vi "MB Slave Write Coils (poly).vi"(1 "Starting Address":u16, 2 "Coils":bool[](array[boolean]), 5 "error in":errorcluster) -> (19 "error out":errorcluster)   [LabVIEW 2023, in "Voegtlin_NI_SMART_Modbus_Drivers.lvlib"]
doc: "Writes multiple coils to the slave memory tables."
uses:
  Voegtlin_NI_SMART_Modbus_Drivers.lvlib
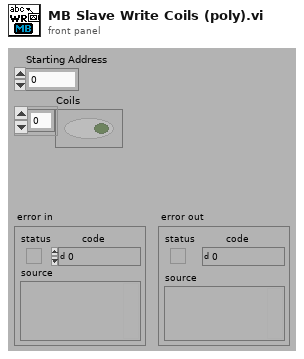
[diagram p1: front panel]
types:
  T1 = enum16{"Discrete Inputs", "Coils", "Input Registers", "Holding Registers"}
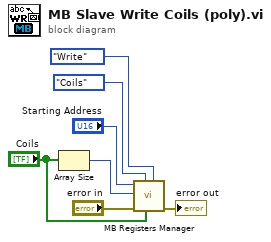
[diagram p0: block diagram]
diagram:
  n1 = Array Size(array="Coils") -> (size(s)=w1:i32)
  n2 = call "MB Registers Manager.vi"("Function"=enum16{"Init", "Read", "Write", "Read All"}."Write", "Bits In"="Coils", "Table"=T1."Coils", "error in (no error)"="error in", "Length"=w1, "Start Address"="Starting Address") -> ("error out"=→"error out":errorcluster)  [unwired: 1 in, 4 out]
